vi "Map.vi"(7 "Action":enum8{"noop", "get", "set", "pop"}(ring), 10 "Timer in":T2, 11 "Timer Id":cluster{"Queue":refnum<queue>, "Message":string}) -> (1 "Found?":bool, 2 "Timer out":T2, 3 "Timers Map":T1(c390))   [LabVIEW 2021, in "QueueTimer.lvlib"]
doc: "Queue timer in memory cache. Queue timers are identified by `<queue>+<timer_message>`.\n\nNote: Timer messages must be unique."
uses:
  QueueTimer.lvlib
  TypeDefs/Timer.ctl
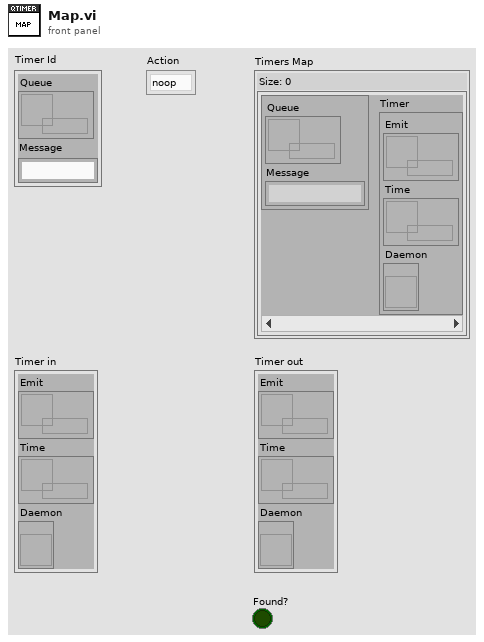
[diagram p1: front panel]
types:
  T1 = map{cluster{"Queue":refnum<queue>, "Message":string}, cluster{"Emit":refnum<queue>, "Time":refnum<data-value>, "Daemon":refnum<vi>}}
  T2 = cluster{"Emit":refnum<queue>, "Time":refnum<data-value>, "Daemon":refnum<vi>}
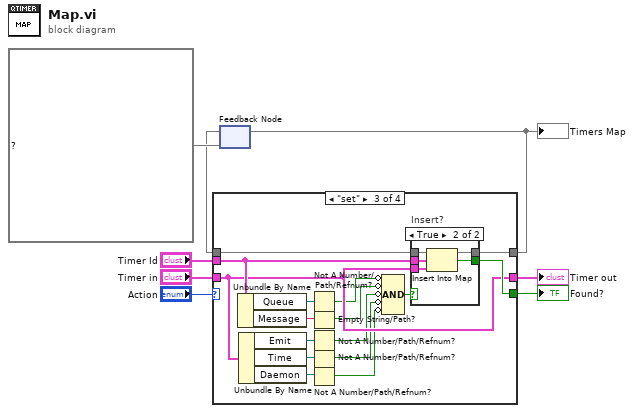
[diagram p0: block diagram]
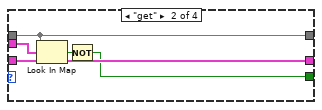
[diagram p3: hidden frame]
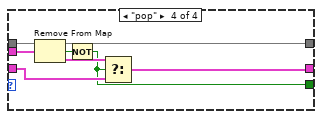
[diagram p5: hidden frame]
diagram:
  n1 = feedback #1(T1 {} ("Timers")) -> (w5:T1)
  n2 = case shown="\"set\"" "Action" {
    tunnel: [w9 w13 w27 w40] -> w8
    tunnel: "Timer Id" -> [_ w14 w28 w44]
    tunnel: w5 -> [w10 w16 w32 w46]
    tunnel: [w10 w16 w31 w45] -> w4
    tunnel: [_ w11 w29 w39] -> w3
    tunnel: "Timer in" -> [w9 w15 w27 w42]
    frame "noop" {
    }
    frame "get" {
      n3 = Look In Map(map=w16, key=w14, default value=w15) -> (key not found?=w12:bool, value=w13:T2)
      n4 = Not(x=w12) -> (.not. x?=w11:bool)
    }
    frame "set" {
      n5 = Unbundle By Name(w28) -> ("Queue"=w24:refnum<queue>, "Message"=w23:string)
      n6 = Unbundle By Name(w27) -> ("Emit"=w26:refnum<queue>, "Time"=w25:refnum<data-value>, "Daemon"=w18:refnum<vi>)
      n7 = Not A Number/Path/Refnum?(number/path/refnum=w24) -> (NaN/Path/Refnum?=w22:bool)
      n8 = Empty String/Path?(string/path=w23) -> (empty?=w21:bool)
      n9 = Not A Number/Path/Refnum?(number/path/refnum=w26) -> (NaN/Path/Refnum?=w20:bool)
      n10 = Not A Number/Path/Refnum?(number/path/refnum=w25) -> (NaN/Path/Refnum?=w19:bool)
      n11 = Not A Number/Path/Refnum?(number/path/refnum=w18) -> (NaN/Path/Refnum?=w17:bool)
      n12 = Compound Arithmetic op=AND(invert w22, invert w21, invert w20, invert w19, invert w17) -> (w30:bool)
      n13 = case "Insert?" shown="True" w30 {
        tunnel: w32 -> [w33 w38]
        tunnel: w27 -> [_ w37]
        tunnel: w28 -> [_ w36]
        tunnel: [w33 w35] -> w31
        tunnel: [_ w34] -> w29
        frame False {
        }
        frame True {
          n14 = Insert Into Map(map in=w38, key=w36, value=w37) -> (map out=w35:T1, key already included?=w34:bool)  [unwired: 1 out]
        }
      }
    }
    frame "pop" {
      n15 = Remove From Map(10:w44, 11:w46) -> (1:w41:T2, 2:w43:bool, 3:w45:T1)
      n16 = Not(x=w43) -> (.not. x?=w39:bool)
      n17 = Select(t=w41, s=w39, f=w42) -> (s? t:f=w40:T2)
    }
  }
  "Timer out" <- w8
  "Found?" <- w3
  "Timers Map" <- w4
  n18 = feedback-in #1(w4) -> ()
